vi "LimitSOC.vi"(5 "Battle Short":bool, 8 "SOC Actual":sgl) -> (0 "Output Low":dbl, 3 "Output High":dbl)   [LabVIEW 2013]
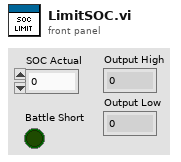
[diagram p1: front panel]
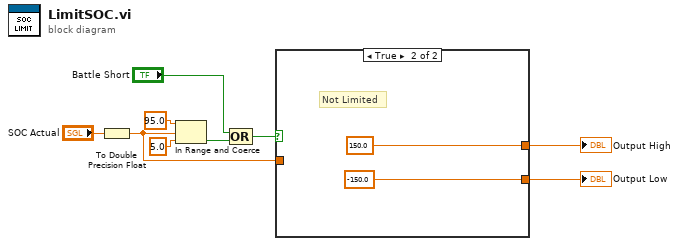
[diagram p0: block diagram]
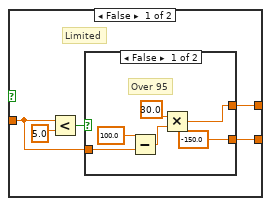
[diagram p2: hidden frame]
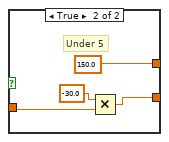
[diagram p3: hidden frame]
diagram:
  n1 = To Double Precision Float(number="SOC Actual") -> (double precision float=w6:dbl)
  n2 = In Range and Coerce(upper limit=95.0, x=w6, lower limit=5.0) -> (In Range?=w3:bool)  [unwired: 1 out]
  n3 = Compound Arithmetic op=OR("Battle Short", w3) -> (w1:bool)
  n4 = case shown="True" w1 {
    tunnel: [w11 150.0 ("Output High")] -> w5
    tunnel: [w12 -150.0 ("Output High")] -> w4
    tunnel: w6 -> [w10 _]
    frame False {
      # "Limited"
      n5 = Less?(x=w10, y=5.0) -> (x < y?=w13:bool)
      n6 = case shown="False" w13 {
        tunnel: [-150.0 w21] -> w12
        tunnel: [w15 150.0 ("y")] -> w11
        tunnel: w10 -> [w16 w22]
        frame False {
          # "Over 95"
          n7 = Subtract(x=100.0, y=w16) -> (x-y=w18:dbl)
          n8 = Multiply(x=30.0, y=w18) -> (x*y=w15:dbl)
        }
        frame True {
          # "Under 5"
          n9 = Multiply(x=-30.0, y=w22) -> (x*y=w21:dbl)
        }
      }
    }
    frame True {
      # "Not Limited"
    }
  }
  "Output High" <- w5
  "Output Low" <- w4
